vi "RunVI.vi"(5 "IP address of target":string, 6 "VI path":path=path "C:/Users/ni-aswcgbld-prod.NI/Desktop/ResourceVIs/TestVIs/timerVI.vi") -> (0 "error out":errorcluster, 1 "array of error description":T1(array[cluster]), 2 "outputs":T3(array[cluster]), 3 "array output?":bool, 4 "Metrics":T2)   [LabVIEW 2019]
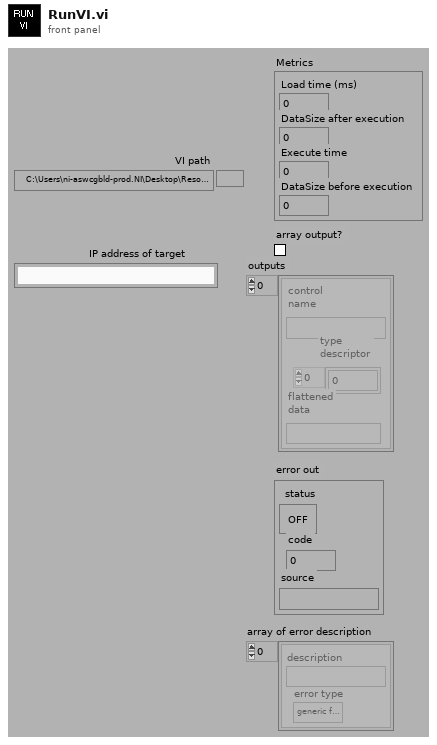
[diagram p1: front panel]
types:
  T1 = cluster{"description":string, "error type":enum32{"generic failure", "boundary case", "precision", "expected error"}}[]
  T2 = cluster{"Load time (ms)":u32, "DataSize after execution":u32, "Execute time":u32, "DataSize before execution":u32}
  T3 = cluster{"control\nname":string, "type\ndescriptor":i16[], "flattened\ndata":string}[]
  T4 = cluster{"description":string, "error type":enum32{"generic failure", "boundary case", "precision", "expected error"}}
  T5 = enum32{"generic failure", "boundary case", "precision", "expected error"}
  T6 = cluster{string, "type string":i16[], "data string":string}
  T7 = cluster{string, "type string":i16[], "data string":string}[]
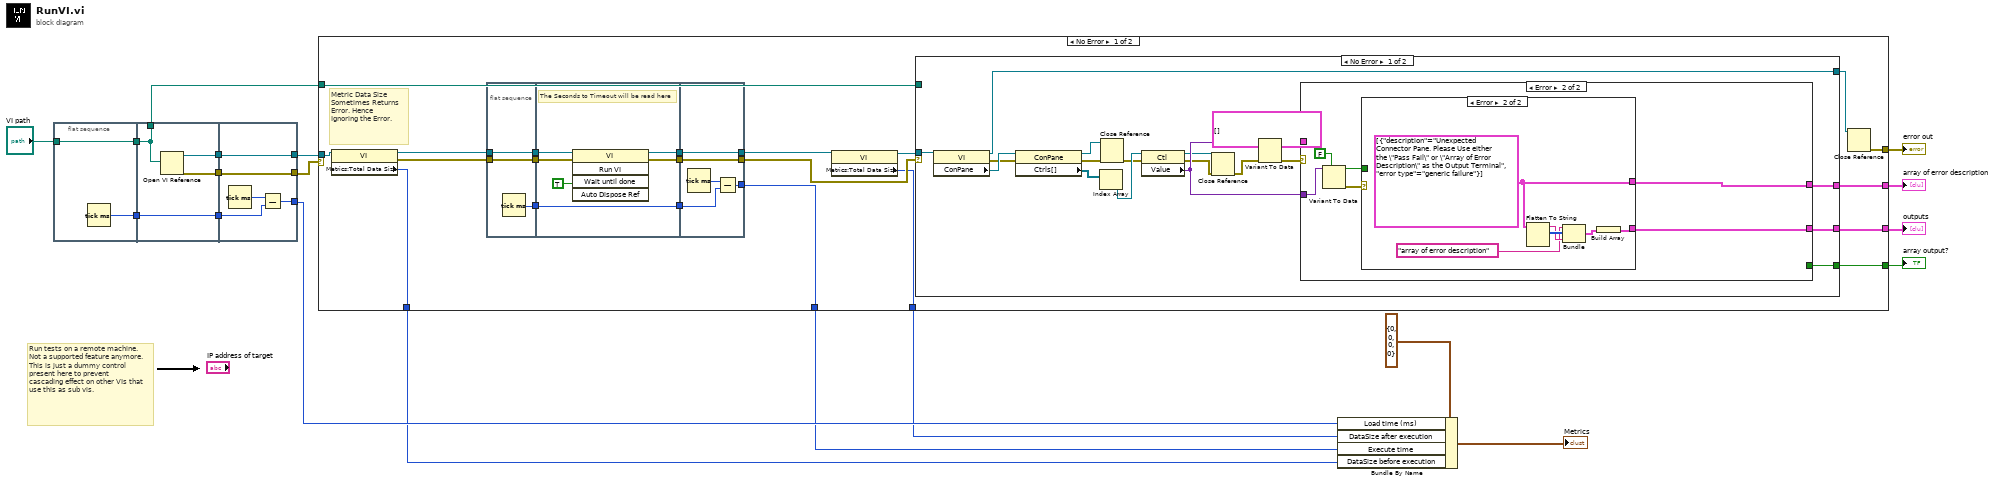
[diagram p0: block diagram]
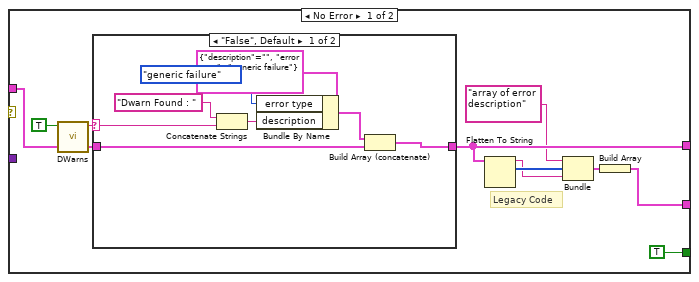
[diagram p2: hidden frame]
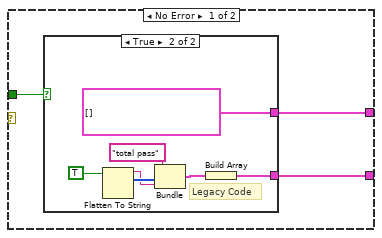
[diagram p4: hidden frame]
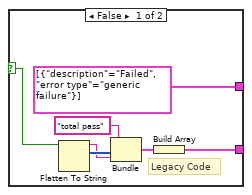
[diagram p5: hidden frame]
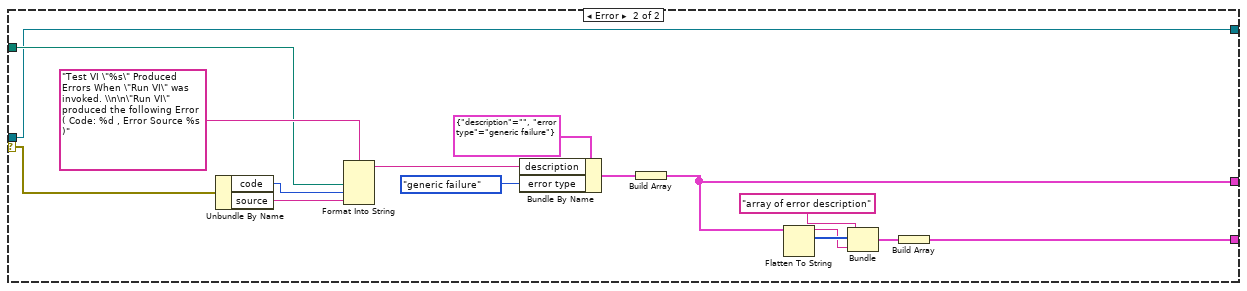
[diagram p6: hidden frame]
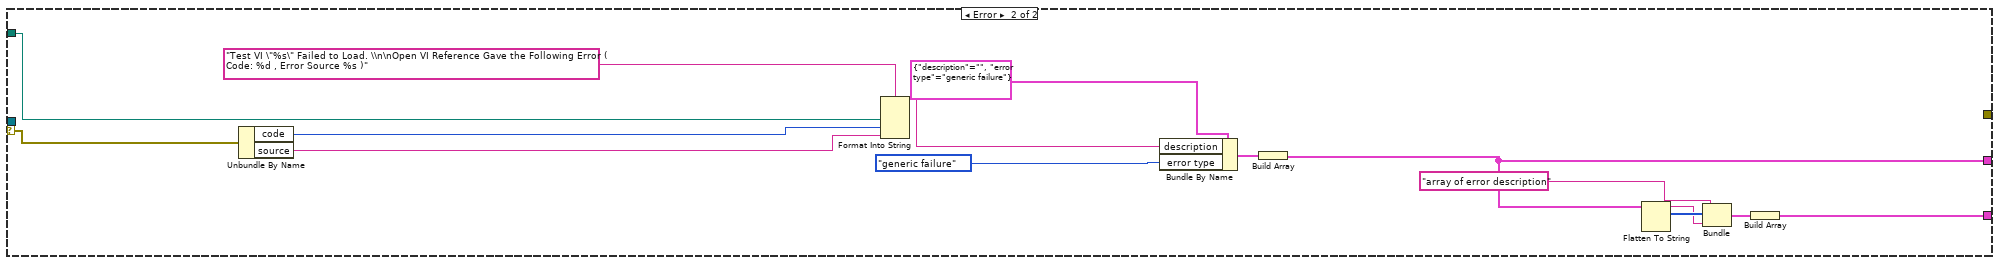
[diagram p7: hidden frame]
diagram:
  # "Run tests on a remote machine. Not a supported feature anymore.\nThis is just a dummy control present here to prevent cascading effect on other VIs that use this as sub vis."
  n1 = flat-sequence {
    tunnel: "VI path" -> [w20]
    tunnel: [w20] -> w13
    tunnel: [w21] -> w12
    tunnel: [w25] -> w11
    tunnel: [w24] -> w10
    tunnel: w13 -> [w22]
    tunnel: w12 -> [w23]
    tunnel: [w23] -> w9
    tunnel: [w22] -> w7
    tunnel: [w27] -> w14
    tunnel: w11 -> [w27]
    tunnel: [w26] -> w8
    tunnel: w10 -> [w26]
    tunnel: [w30] -> w19
    tunnel: w9 -> [w28]
    frame #0 {
      n2 = Tick Count (ms)() -> (millisecond timer value=w21:u32)
    }
    frame #1 {
      n3 = Open VI Reference(vi path=w22) -> (vi reference=w25:refnum<vi>, error out=w24:errorcluster)  [unwired: 1 in, 4 out]
    }
    frame #2 {
      n4 = Tick Count (ms)() -> (millisecond timer value=w29:u32)
      n5 = Subtract(x=w29, y=w28) -> (x-y=w30:u32)
    }
  }
  n6 = case shown="No Error" w8 {
    selector: w8 -> [_ w161]
    tunnel: [w51 _] -> w18
    tunnel: w14 -> [w50 _]
    tunnel: w7 -> [w40 w162]
    tunnel: [w42 w150] -> w4
    tunnel: [w43 _] -> w6
    tunnel: [w36 _] -> w5
    tunnel: [w35 w149] -> w3
    tunnel: [w33 _] -> w2
    tunnel: [w32 _] -> w1
    frame No Error {
      # "Metric Data Size Sometimes Returns Error. Hence Ignoring the Error."
      n7 = property class="VI"(reference=w50) -> (reference out=w49:refnum<vi>, error out=w41:errorcluster, "Metrics:Total Data Size"=w51:u32)  [unwired: 1 in]
      n8 = flat-sequence {
        tunnel: w49 -> [w54]
        tunnel: [w54] -> w48
        tunnel: [w53] -> w44
        tunnel: w41 -> [w52]
        tunnel: [w52] -> w31
        tunnel: w48 -> [w58]
        tunnel: [w57] -> w47
        tunnel: [w56] -> w46
        tunnel: [w60] -> w45
        tunnel: w44 -> [w60]
        tunnel: w31 -> [w55]
        tunnel: [w64] -> w37
        tunnel: [w65] -> w39
        tunnel: w47 -> [w65]
        tunnel: w46 -> [w64]
        tunnel: w45 -> [w62]
        tunnel: [w61] -> w43
        frame #0 {
          n9 = Tick Count (ms)() -> (millisecond timer value=w53:u32)
        }
        frame #1 {
          # "The Seconds to Timeout will be read here"
          n10 = invoke class="VI" method="Run VI"(reference=w58, error in=w55, "Wait until done"=TRUE ("Wait Until Done")) -> (reference out=w57:refnum<vi>, error out=w56:errorcluster)  [unwired: 2 in, 3 out]
        }
        frame #2 {
          n11 = Tick Count (ms)() -> (millisecond timer value=w63:u32)
          n12 = Subtract(x=w63, y=w62) -> (x-y=w61:u32)
        }
      }
      n13 = property class="VI"(reference=w39) -> (reference out=w38:refnum<vi>, "Metrics:Total Data Size"=w36:u32)  [unwired: 1 in, 1 out]
      n14 = case shown="No Error" w37 {
        selector: w37 -> [_ w140]
        tunnel: w38 -> [w81 w133]
        tunnel: [w78 w135] -> w42
        tunnel: w40 -> [_ w141]
        tunnel: [w74 w134] -> w35
        tunnel: [w73 w133] -> w34
        tunnel: [w72 _] -> w33
        frame No Error {
          n15 = property class="VI"(reference=w81) -> (reference out=w73:refnum<vi>, error out=w77:errorcluster, "ConPane"=w84:refnum<vi>)  [unwired: 1 in]
          n16 = property class="ConPane"(reference=w84, error in=w77) -> (reference out=w71:refnum<vi>, error out=w70:errorcluster, "Ctrls[]"=w83:refnum<vi>[])
          n17 = Index Array(array=w83) -> (element=w82:refnum<vi>)  [unwired: 1 in]
          n18 = Close Reference(reference=w71, error in (no error)=w70) -> (error out=w69:errorcluster)
          n19 = property class="Ctl"(reference=w82, error in=w69) -> (reference out=w66:refnum<vi>, error out=w68:errorcluster, "Value"=w75:variant)
          n20 = Close Reference(reference=w66, error in (no error)=w68) -> (error out=w67:errorcluster)
          n21 = Variant To Data(error in=w67, type=T1 [] ("array of error description"), Variant=w75) -> (data=w76:T1, error out=w79:errorcluster)
          n22 = case shown="Error" w79 {
            tunnel: w75 -> [_ w109]
            tunnel: [w89 w106] -> w78
            tunnel: w76 -> [w92 _]
            tunnel: [w86 w104] -> w74
            tunnel: [TRUE _] -> w72
            frame No Error {
              # "Legacy Code"
              n23 = call "DWarns.vi"("End Caching (false)"=TRUE) -> ("DWarn Buffer"=w93:string)  [unwired: 10 out]
              n24 = case shown="\"False\", Default" w93 {
                selector: w93 -> [w99 _]
                tunnel: w92 -> [w96 w103]
                tunnel: [w95 w103] -> w89
                frame "False", Default {
                  n25 = Concatenate Strings("Dwarn Found : " ("string"), w99) -> (w102:string)
                  n26 = Bundle By Name(cluster=T4 {"description"="", "error type"=enum."generic failure"} ("error description"), "error type"=T5."generic failure", "description"=w102) -> (w98:T4)
                  n27 = Build Array (concatenate)(w98, w96) -> (w95:T1)
                }
                frame "" {
                }
              }
              n28 = Flatten To String(anything=w89) -> (data string=w87:string, type string=w91:i16[])  [unwired: 1 in, 3 out]
              n29 = Bundle("array of error description", "type string"=w91, "data string"=w87) -> (w90:T6)  [unwired: 1 out]
              n30 = Build Array(w90) -> (w86:T7)
            }
            frame Error {
              n31 = Variant To Data(type=FALSE ("total pass"), Variant=w109) -> (data=w107:bool, error out=w105:errorcluster)  [unwired: 1 in]
              n32 = case shown="Error" w105 {
                tunnel: w107 -> [w112 _]
                tunnel: [w111 w131] -> w106
                tunnel: [w110 w128] -> w104
                frame No Error {
                  n33 = case shown="True" w112 {
                    selector: w112 -> [w114 _]
                    tunnel: [T1 [{"description"="Failed", "error type"=enum."generic failure"}] ("array of error description") T1 [] ("array of error description")] -> w111
                    tunnel: [w113 w120] -> w110
                    frame False {
                      # "Legacy Code"
                      n34 = Flatten To String(anything=w114) -> (data string=w116:string, type string=w117:i16[])  [unwired: 1 in, 3 out]
                      n35 = Bundle("total pass", "type string"=w117, "data string"=w116) -> (w115:T6)  [unwired: 1 out]
                      n36 = Build Array(w115) -> (w113:T7)
                    }
                    frame True {
                      # "Legacy Code"
                      n37 = Flatten To String(anything=TRUE) -> (data string=w123:string, type string=w124:i16[])  [unwired: 1 in, 3 out]
                      n38 = Bundle("total pass", "type string"=w124, "data string"=w123) -> (w122:T6)  [unwired: 1 out]
                      n39 = Build Array(w122) -> (w120:T7)
                    }
                  }
                }
                frame Error {
                  w131 = T1 [{"description"="Unexpected Connector Pane. Please Use either the \"Pass Fail\" or \"Array of Error Description\" as the Output Terminal", "error type"=enum."generic failure"}] ("array of error description")
                  n40 = Flatten To String(anything=w131) -> (data string=w130:string, type string=w132:i16[])  [unwired: 1 in, 3 out]
                  n41 = Bundle("array of error description", "type string"=w132, "data string"=w130) -> (w127:T6)  [unwired: 1 out]
                  n42 = Build Array(w127) -> (w128:T7)
                }
              }
            }
          }
        }
        frame Error {
          n43 = Unbundle By Name(w140) -> ("code"=w147:i32, "source"=w146:string)
          n44 = Format Into String(format string="Test VI \"%s\" Produced Errors When \"Run VI\" was invoked. \\n\n\"Run VI\" produced the following Error ( Code: %d , Error Source %s )" ("description"), w141, w147, w146) -> (resulting string=w143:string)  [unwired: 2 in, 1 out]
          n45 = Bundle By Name(cluster=T4 {"description"="", "error type"=enum."generic failure"} ("error description"), "description"=w143, "error type"=T5."generic failure") -> (w142:T4)
          n46 = Build Array(w142) -> (w135:T1)
          n47 = Flatten To String(anything=w135) -> (data string=w137:string, type string=w138:i16[])  [unwired: 1 in, 3 out]
          n48 = Bundle("array of error description", "type string"=w138, "data string"=w137) -> (w136:T6)  [unwired: 1 out]
          n49 = Build Array(w136) -> (w134:T7)
        }
      }
      n50 = Close Reference(reference=w34) -> (error out=w32:errorcluster)  [unwired: 1 in]
    }
    frame Error {
      n51 = Unbundle By Name(w161) -> ("code"=w160:i32, "source"=w159:string)
      n52 = Format Into String(format string="Test VI \"%s\" Failed to Load. \\n\nOpen VI Reference Gave the Following Error ( Code: %d , Error Source %s )" ("description"), w162, w160, w159) -> (resulting string=w156:string)  [unwired: 2 in, 1 out]
      n53 = Bundle By Name(cluster=T4 {"description"="", "error type"=enum."generic failure"} ("error description"), "description"=w156, "error type"=T5."generic failure") -> (w155:T4)
      n54 = Build Array(w155) -> (w150:T1)
      n55 = Flatten To String(anything=w150) -> (data string=w152:string, type string=w153:i16[])  [unwired: 1 in, 3 out]
      n56 = Bundle("array of error description", "type string"=w153, "data string"=w152) -> (w151:T6)  [unwired: 1 out]
      n57 = Build Array(w151) -> (w149:T7)
    }
  }
  "outputs" <- w3
  "error out" <- w1
  "array output?" <- w2
  "array of error description" <- w4
  n58 = Bundle By Name(cluster=T2 {"Load time (ms)"=0, "DataSize after execution"=0, "Execute time"=0, "DataSize before execution"=0} ("Metrics"), "Load time (ms)"=w19, "DataSize after execution"=w5, "Execute time"=w6, "DataSize before execution"=w18) -> (→"Metrics":T2)
